vi "PI_V.vi"(10 "PicamValueType":T2, 11 "PicamConstraintType":T3) -> (3 "PicamParameter value":u32)   [LabVIEW 2019, in "PICam.lvlib"]
uses:
  PICam.lvlib
  types/PicamConstraintType.ctl
  types/PicamValueType.ctl
panel:
  in  "PicamParameter":T1(ring)
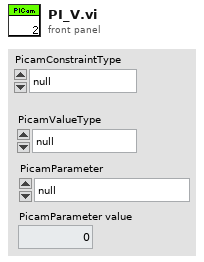
[diagram p1: front panel]
types:
  T1 = enum32{"null", "AcitveWidth", "ActiveHeight", "ActiveLeftMargin", "ActiveTopMargin", "ActiveRightMargin", "ActiveBottomMargin", "SensorTemperatureReading", ""}
  T2 = typedef "PicamValueType.ctl" = enum32{"null", "LargeInteger", "FloatingPoint", "Rois", "Pulse", "Modulations"}
  T3 = typedef "PicamConstraintType.ctl" = enum32{"null", "None", "Range", "Collection", "Rois", "Pulse", "Modulations"}
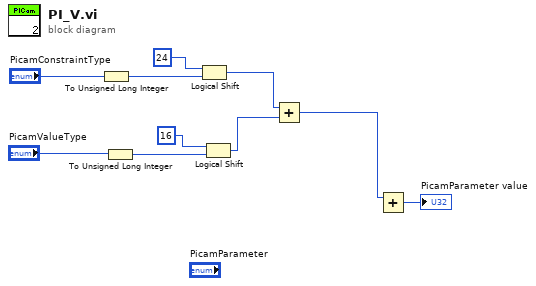
[diagram p0: block diagram]
diagram:
  n1 = To Unsigned Long Integer(number="PicamConstraintType") -> (unsigned 32bit integer=w9:u32)
  n2 = To Unsigned Long Integer(number="PicamValueType") -> (unsigned 32bit integer=w8:u32)
  n3 = Logical Shift(y=u32 24, x=w9) -> (x << y=w5:u32)
  n4 = Logical Shift(y=u32 16, x=w8) -> (x << y=w4:u32)
  n5 = Add(x=w5, y=w4) -> (x+y=w3:u32)
  n6 = Add(x=w3) -> (y=w2:u32, x+y=→"PicamParameter value":u32)
